vi "Enqeue with Display Update.vi"(7 "Display Message":string, 8 "error in":errorcluster, 9 "Data":variant, 10 "Message":string) -> (0 "error out":errorcluster)   [LabVIEW 2024, in "User Interface Control.lvlib"]
uses:
  User Interface Control.lvlib
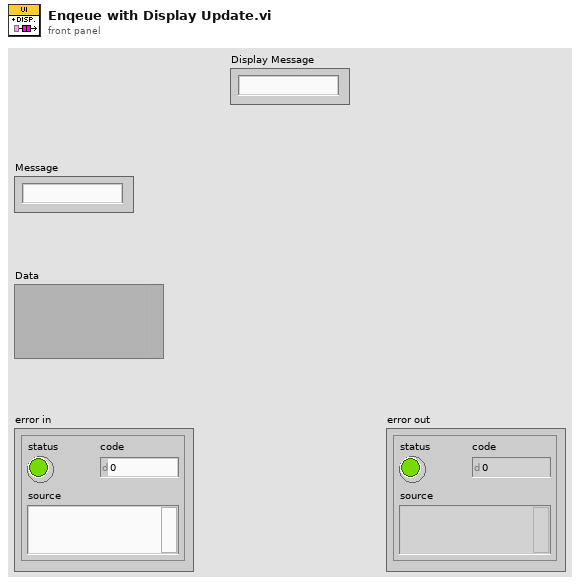
[diagram p1: front panel]
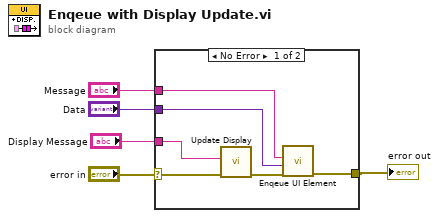
[diagram p0: block diagram]
diagram:
  n1 = case shown="No Error" "error in" {
    selector: "error in" -> [w11 w12]
    tunnel: "Message" -> [w6 _]
    tunnel: "Data" -> [w7 _]
    tunnel: [w9 w12] -> w5
    tunnel: "Display Message" -> [w8 _]
    frame No Error {
      n2 = call "Update Display.vi"("error in"=w11, "Display Message"=w8) -> ("error out"=w10:errorcluster)  [unwired: 9 in]
      n3 = call "Enqeue UI Element.vi"("error in"=w10, "Data"=w7, "Message"=w6) -> ("error out"=w9:errorcluster)  [unwired: 8 in]
    }
    frame Error {
    }
  }
  "error out" <- w5
